vi "Load Technique.vi"(4 "Last Protocol":bool=TRUE, 5 "Display Parameters?":bool, 6 "First Protocol":bool=TRUE, 7 "TechniqueParameters":T2[](array[typedef])=[{"String Label"="1_Tc_lim", "Type"=0, "Valeur"=0, "Index"=0}], 8 "error in (no error)":errorcluster, 9 "Parameters":T1, 10 "Selected Channel":u8=6, 11 "ID In":i32) -> (0 "error out":errorcluster, 1 "Fichier .ecc":string, 3 "ID  Out":i32)   [LabVIEW 2022 SP3, in "EClib functions.lvlib"]
doc: "This VI loads protocol in the selected channel."
uses:
  EClib functions.lvlib
  TechniqueParameters.ctl
  Parameters.ctl
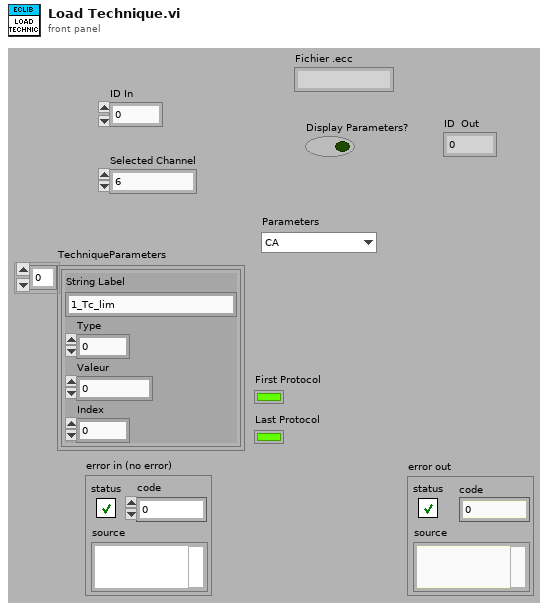
[diagram p1: front panel]
types:
  T1 = typedef "EClib functions.lvlib/Parameters.ctl" = enum16{"CA", "CASG", "CP", "GEIS", "ISCAN", "OCV", "PEIS", "SCCX", "SGEIS", "SPEIS", "VSCAN", "MP"}
  T2 = typedef "EClib functions.lvlib/TechniqueParameters.ctl" = cluster{"String Label":string, "Type":i32, "Valeur":i32, "Index":i32}
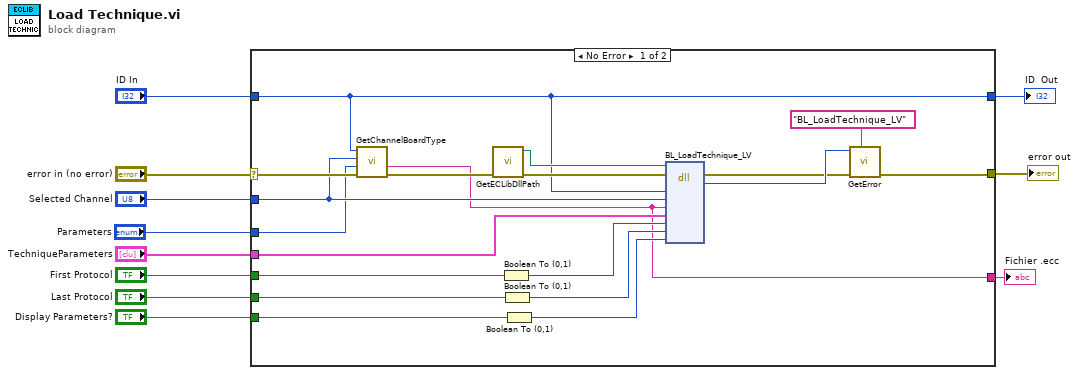
[diagram p0: block diagram]
diagram:
  n1 = case shown="No Error" "error in (no error)" {
    selector: "error in (no error)" -> [w17 w32]
    tunnel: [w26 w32] -> w10
    tunnel: "ID In" -> [w15 w31]
    tunnel: [w15 w31] -> w8
    tunnel: "Selected Channel" -> [w14 _]
    tunnel: "TechniqueParameters" -> [w23 _]
    tunnel: "First Protocol" -> [w22 _]
    tunnel: "Last Protocol" -> [w21 _]
    tunnel: "Display Parameters?" -> [w18 _]
    tunnel: "Parameters" -> [w13 _]
    tunnel: [w12 _] -> w1
    frame No Error {
      n2 = call "GetChannelBoardType.vi"("error in (no error)"=w17, "Parameters"=w13, "Channel"=w14, "ConnectionID IN"=w15) -> ("error out"=w16:errorcluster, "Fichier .ecc"=w12:string)  [unwired: 4 in, 2 out]
      n3 = call "GetECLibDllPath.vi"("error in (no error)"=w16) -> ("error out"=w20:errorcluster, "ECLibDLLPath"=w27:path)  [unwired: 9 in]
      n4 = Boolean To (0,1)(Boolean=w22) -> (0, 1=w30:i16)
      n5 = Boolean To (0,1)(Boolean=w21) -> (0, 1=w29:i16)
      n6 = Boolean To (0,1)(Boolean=w18) -> (0, 1=w28:i16)
      n7 = dll-call lib="?" fn="BL_LoadTechnique_LV"(path in=w27, error in=w20, "arg1"=w15, "arg2"=w14, "arg3"=w12, "arg4"=w23, "arg5"=w30, "arg6"=w29, "arg7"=w28) -> (error out=w19:errorcluster, "return type"=w24:i32)  [unwired: 8 in, 1 out]
      n8 = call "GetError.vi"("DLLFunction"="BL_LoadTechnique_LV", "error in"=w19, "code"=w24) -> ("error out"=w26:errorcluster)  [unwired: 8 in]
    }
    frame Error {
    }
  }
  "error out" <- w10
  "ID  Out" <- w8
  "Fichier .ecc" <- w1
